vi "read adxl tri.vi"(7 "file path":path, 8 "name or relative path":string="Craig walking ADI.csv") -> (0 "sensor 3 acceleration":dbl[][](array[numeric]), 1 "sensor 2 acceleration":dbl[][](array[numeric]), 2 "sensor 1 acceleration":dbl[][](array[numeric]), 3 "Frequency (Hz)":dbl)   [LabVIEW 2009]
uses:
  <vilib>/Utility/file.llb/Read From Spreadsheet File (DBL).vi
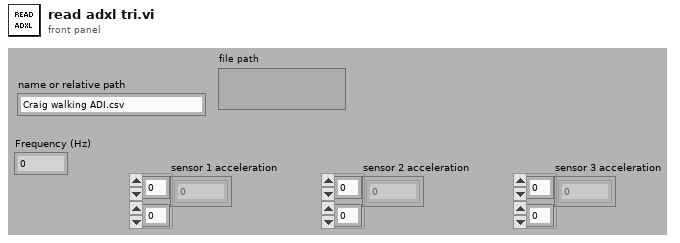
[diagram p1: front panel]
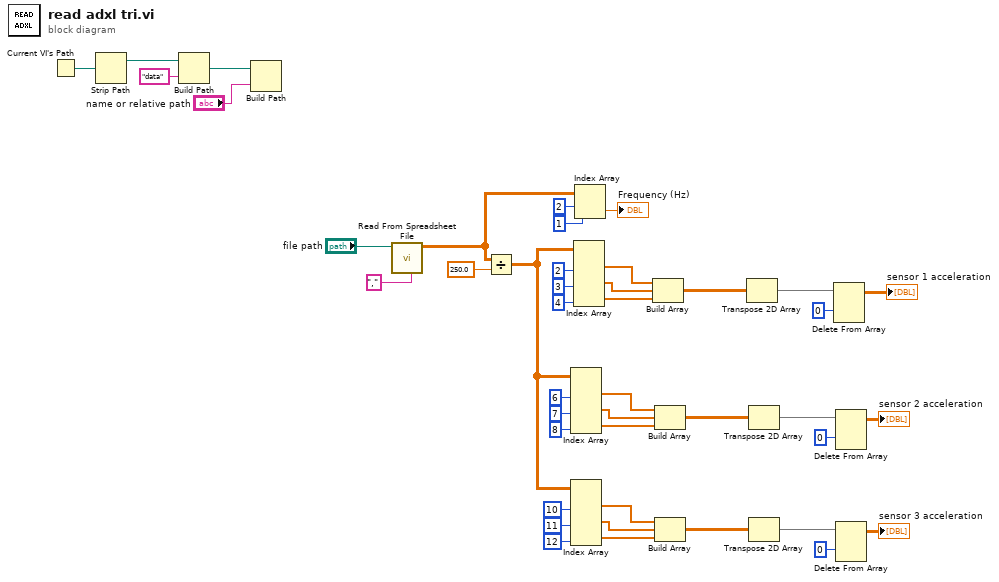
[diagram p0: block diagram]
diagram:
  n1 = Current VI's Path() -> (path=w42:path)
  n2 = Strip Path(path=w42) -> (stripped path=w40:path)  [unwired: 1 out]
  n3 = Build Path(base path=w40, name or relative path="data") -> (appended path=w39:path)
  n4 = Build Path(base path=w39, name or relative path="name or relative path") -> ()  [unwired: 1 out]
  n5 = call-poly <vilib>:"Read From Spreadsheet File.vi"("delimiter (\\t)"="," ("delimiter (\\t)"), "file path (dialog if empty)"="file path") -> ("all rows"=w2:dbl[][])  [unwired: 5 in, 4 out]
  n6 = Divide(x=w2, y=250.0) -> (x/y=w3:dbl[][])
  n7 = Index Array(array=w3, index (col) #1=6 ("disabled index (col)"), index (col) #2=7 ("index (col)"), index (col) #3=8 ("index (col)")) -> (element #1=w17:dbl[], element #2=w18:dbl[], element #3=w19:dbl[])  [unwired: 3 in]
  n8 = Index Array(array=w3, index (col) #1=10 ("disabled index (col)"), index (col) #2=11 ("index (col)"), index (col) #3=12 ("index (col)")) -> (element #1=w7:dbl[], element #2=w8:dbl[], element #3=w9:dbl[])  [unwired: 3 in]
  n9 = Index Array(array=w3, index (col) #1=2 ("disabled index (col)"), index (col) #2=3 ("index (col)"), index (col) #3=4 ("index (col)")) -> (element #1=w31:dbl[], element #2=w30:dbl[], element #3=w29:dbl[])  [unwired: 3 in]
  n10 = Index Array(array=w2, index (row)=2, index (col)=1 ("disabled index (col)")) -> (element=→"Frequency (Hz)":dbl)
  n11 = Build Array(w31, w30, w29) -> (w28:dbl[][])
  n12 = Build Array(w17, w18, w19) -> (w22:dbl[][])
  n13 = Build Array(w7, w8, w9) -> (w12:dbl[][])
  n14 = Transpose 2D Array(2D array=w28) -> (transposed array=w27:dbl[][])
  n15 = Transpose 2D Array(2D array=w22) -> (transposed array=w21:dbl[][])
  n16 = Transpose 2D Array(2D array=w12) -> (transposed array=w11:dbl[][])
  n17 = Delete From Array(array=w27, index (row)=0) -> (array with subset deleted=→"sensor 1 acceleration":dbl[][])  [unwired: 2 in, 1 out]
  n18 = Delete From Array(array=w21, index (row)=0) -> (array with subset deleted=→"sensor 2 acceleration":dbl[][])  [unwired: 2 in, 1 out]
  n19 = Delete From Array(array=w11, index (row)=0) -> (array with subset deleted=→"sensor 3 acceleration":dbl[][])  [unwired: 2 in, 1 out]
